vi "TriggerRateCalculator.vi"(10 "Count":i32) -> (2 "rep rate":dbl)   [LabVIEW 2013]
uses:
  <vilib>/ptbypt/NI_PtbyPt.lvlib
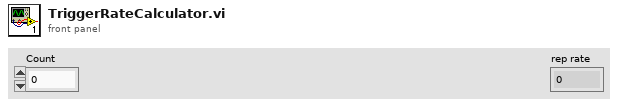
[diagram p1: front panel]
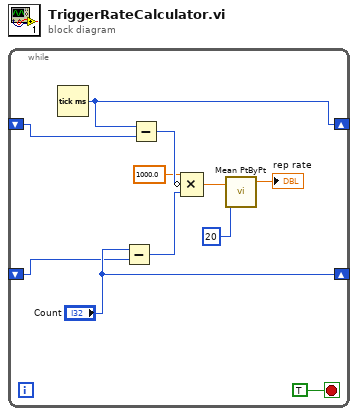
[diagram p0: block diagram]
diagram:
  n1 = while {
    shift-right: ["Count"] -> _
    shift-left: _ -> [w1]
    shift-right: [w10] -> _
    shift-left: _ -> [w2]
    stop <- TRUE stop-if-true
    n2 = Tick Count (ms)() -> (millisecond timer value=w10:u32)
    n3 = Subtract(x="Count", y=w1) -> (x-y=w7:i32)
    n4 = Subtract(x=w10, y=w2) -> (x-y=w9:u32)
    n5 = Compound Arithmetic op=MULTIPLY(1000.0, invert w9, w7) -> (w6:dbl)
    n6 = call <vilib>:"Mean PtByPt.vi"("x"=w6, "sample length"=20) -> ("mean"=→"rep rate":dbl)  [unwired: 2 in, 1 out]
  }
